vi "Addon.Version.Upgrade.vi"(8 "error in (no error)":errorcluster, 11 "Device Item Ref in in":T1 format="%.0x") -> (0 "error out":errorcluster, 3 "Device Item Ref out":T1 format="%.0x")   [LabVIEW 2025, in "Protection and Counter Addon Shared.lvlib"]
uses:
  Protection and Counter Addon Shared.lvlib
  <vilib>/NI VeriStand/Custom Device API/Custom Device Item Ref.ctl
  <vilib>/NI VeriStand/Custom Device API/Custom Device Channel.ctl
  <vilib>/NI VeriStand/Custom Device API/Custom Device Channel Type.ctl
  GUID Lookup.vi
  <vilib>/NI/NI VeriStand Advanced SysDef API/_SubVIs/SysDef.Search.GUID.vi
  <vilib>/NI/NI VeriStand Advanced SysDef API/_SubVIs/SysDef.Search.GUIDs.vi
  <vilib>/NI/NI VeriStand Advanced SysDef API/_SubVIs/SysDef.Search.Parent.vi
  NationalInstruments.VeriStand.SystemDefinitionAPI
  <vilib>/NI/NI VeriStand Advanced SysDef API/SysDef API/Advanced System Definition.lvlib
  <vilib>/NI VeriStand/Custom Device API/Custom Device API.lvlib
  SubModules/Frame-Protection-Support/Source/System Explorer/Protection and Counter Support System Explorer.lvlib
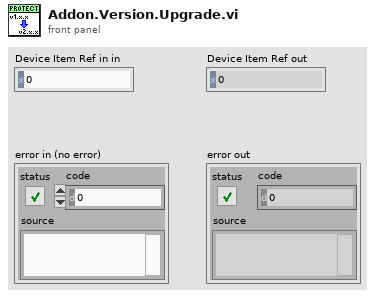
[diagram p1: front panel]
types:
  T1 = typedef "Custom Device API.lvlib/Custom Device Item Ref.ctl" = u64
  T2 = typedef "Custom Device API.lvlib/Custom Device Channel.ctl" = cluster{"Type":T3, "Units":string, "Default Value":dbl, "Faultable":bool, "Scalable":bool}
  T3 = typedef "Custom Device API.lvlib/Custom Device Channel Type.ctl" = enum16{"Input", "Output"}
  T4 = typedef "Protection and Counter Support System Explorer.lvlib/Protection Signal Settings.ctl" = cluster{"Input Channels":T5[], "Protection Type":T6}
  T5 = typedef "Protection and Counter Support System Explorer.lvlib/Protection Signal Linked Channel.ctl" = cluster{"Node Ref":T1}
  T6 = typedef "Protection and Counter Support Shared.lvlib/Protection Type.ctl" = enum16{"Arb ID + Bytes Checksum with Inversion", "Arb ID + Bytes CRC with Inversion", "Reversed Raw Signal Checksum with Inversion", "Concatenated Two's Compliment"}
  T7 = typedef "Advanced System Definition.lvlib/TreeItem.Info.ctl" = cluster{"Name":string, "Description":string, "GUID":string, "Is Channel":bool, "Channel":T2, "Is Waveform":bool, "Waveform":T8}
  T8 = typedef "Custom Device API.lvlib/Custom Device Waveform.ctl" = cluster{"Data Type":T9, "Units":string}
  T9 = typedef "Custom Device API.lvlib/Custom Device Waveform DataType.ctl" = enum16{"Double", "Complex Double"}
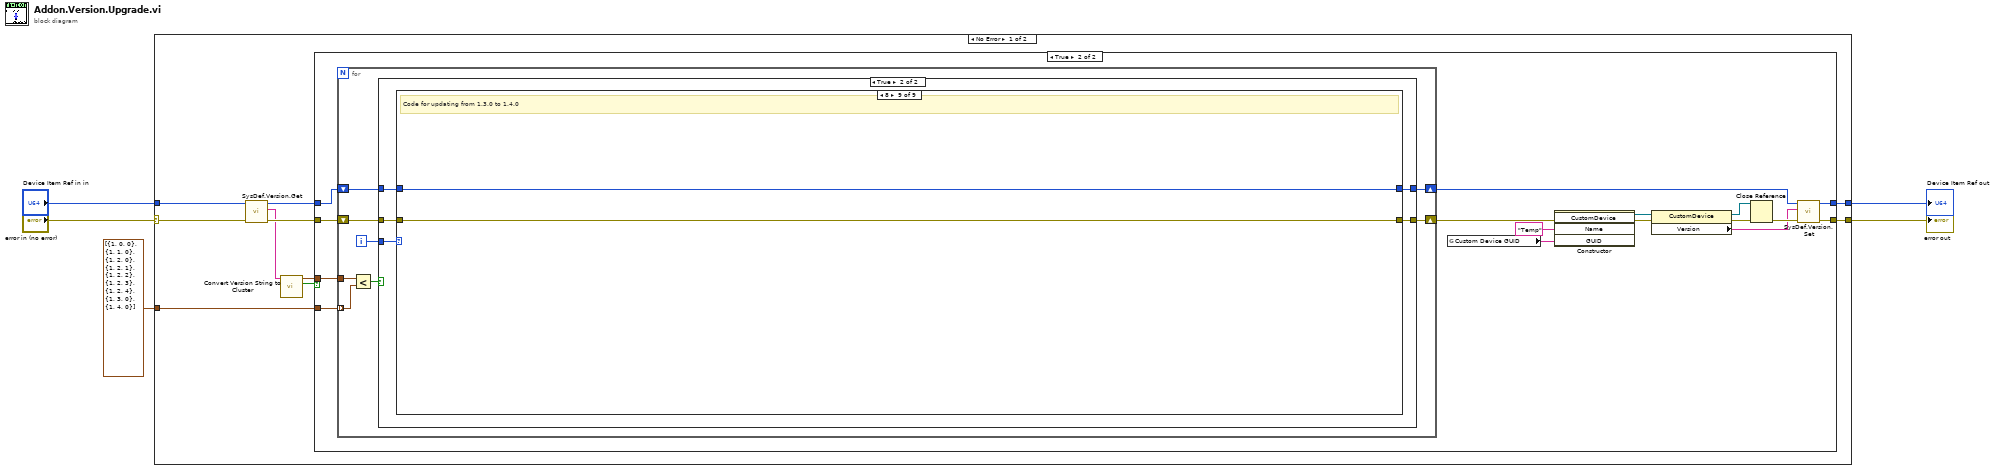
[diagram p0: block diagram]
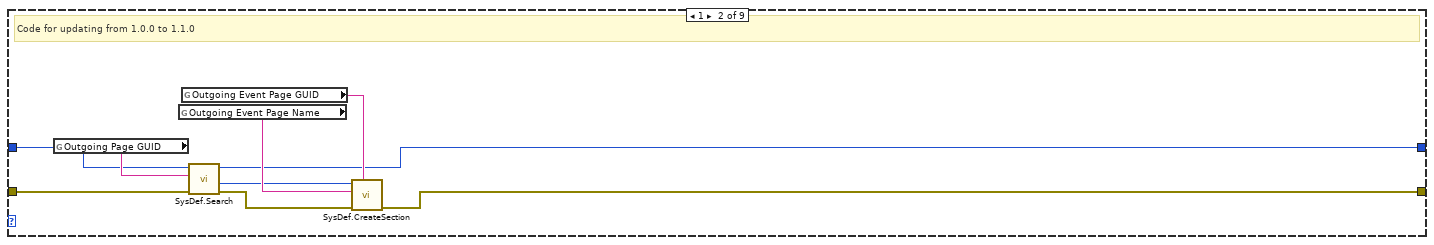
[diagram p5: hidden frame]
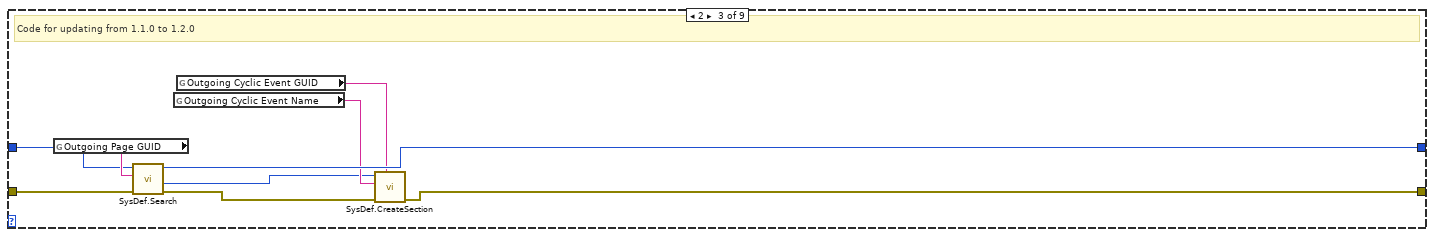
[diagram p6: hidden frame]
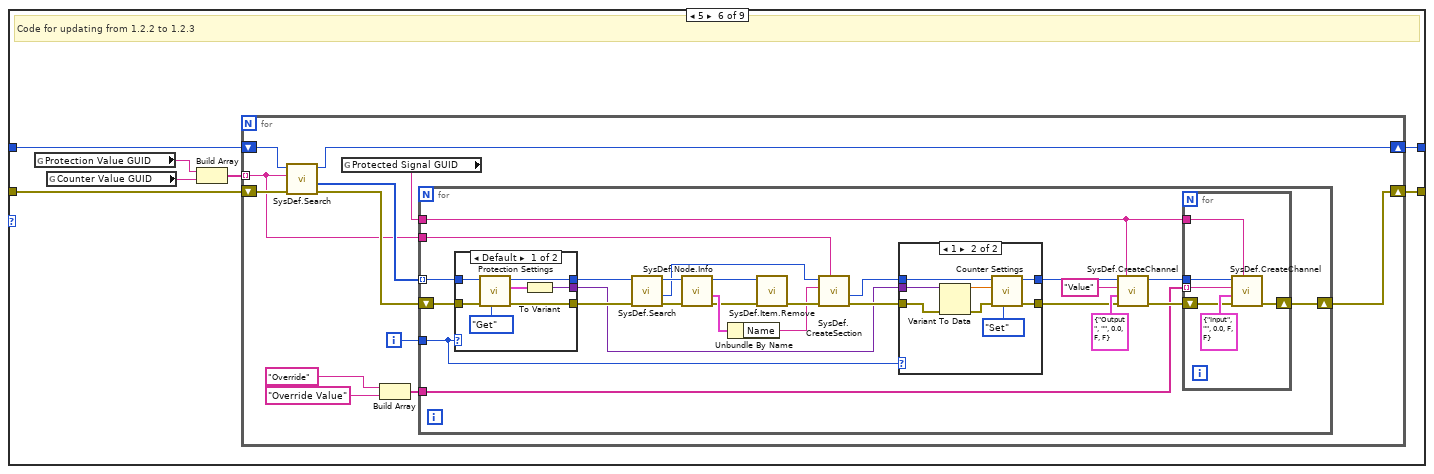
[diagram p9: hidden frame]
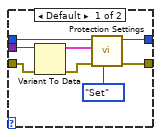
[diagram p10: hidden frame]
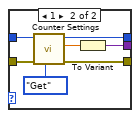
[diagram p11: hidden frame]
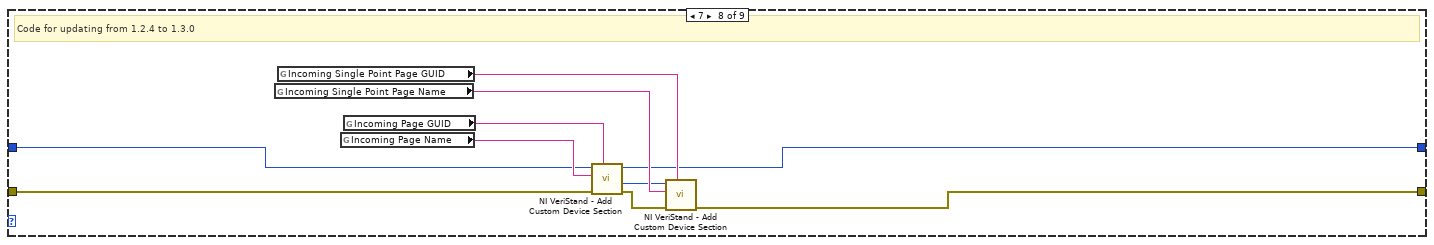
[diagram p13: hidden frame]
diagram:
  n1 = case shown="No Error" "error in (no error)" {
    selector: "error in (no error)" -> [w12 w169]
    tunnel: [w14 w169] -> w2
    tunnel: "Device Item Ref in in" -> [w11 w168]
    tunnel: [w13 w168] -> w4
    tunnel: cluster{i32, i32, i32}[] [{1, 0, 0}, {1, 1, 0}, {1, 2, 0}, {1, 2, 1}, {1, 2, 2}, {1, 2, 3}, {1, 2, 4}, {1, 3, 0}, {1, 4, 0}] -> [w15 _]
    frame No Error {
      n2 = call <vilib>:"SysDef.Version.Get.vi"("error in (no error)"=w12, "nodeID"=w11) -> ("error out"=w10:errorcluster, "Version"=w8:string, "nodeID out"=w9:u64)  [unwired: 7 in]
      n3 = call "Convert Version String to Cluster.vi"("Version"=w8) -> ("Version Valid?"=w6:bool, "Version"=w7:cluster{i32, i32, i32})  [unwired: 9 in]
      n4 = case shown="True" w6 {
        tunnel: w15 -> [_ w25]
        tunnel: [w16 w23] -> w14
        tunnel: [w17 w21] -> w13
        tunnel: w10 -> [w16 w20]
        tunnel: w9 -> [w17 w19]
        tunnel: w7 -> [_ w18]
        frame False {
        }
        frame True {
          n5 = for {
            tunnel: w25 -> [w36] mode=indexing
            shift-right: [w40] -> w24
            shift-left: w20 -> [w34]
            shift-right: [w39] -> w26
            shift-left: w19 -> [w35]
            tunnel: w18 -> [w37]
            i -> [w38]
            n6 = Less?(x=w37, y=w36) -> (x < y?=w41:bool)
            n7 = case shown="True" w41 {
              tunnel: w34 -> [w43 w48]
              tunnel: w35 -> [w42 w47]
              tunnel: [w43 w45] -> w40
              tunnel: [w42 w46] -> w39
              tunnel: w38 -> [_ w44]
              frame False {
              }
              frame True {
                n8 = case shown="8" w44 {
                  tunnel: w48 -> [w49 w56 w67 w69 w71 w78 w154 w158 w167]
                  tunnel: w47 -> [w50 w55 w66 w70 w72 w73 w155 w159 w166]
                  tunnel: [w50 w52 w65 w70 w72 w79 w155 w157 w166] -> w46
                  tunnel: [w49 w51 w62 w69 w71 w77 w154 w156 w167] -> w45
                  frame Default {
                  }
                  frame 1 {
                    # "Code for updating from 1.0.0 to 1.1.0"
                    n9 = global read "GUID Lookup.vi" "Outgoing Page GUID"() -> (w57:string)
                    n10 = global read "GUID Lookup.vi" "Outgoing Event Page Name"() -> (w59:string)
                    n11 = global read "GUID Lookup.vi" "Outgoing Event Page GUID"() -> (w58:string)
                    n12 = call-poly <vilib>:"SysDef.Search.vi"("error in (no error)"=w56, "GUID"=w57, "nodeID"=w55) -> ("error out"=w54:errorcluster, "Value out"=w53:u64, "nodeID out"=w52:u64)  [unwired: 5 in, 1 out]
                    n13 = call <vilib>:"SysDef.CreateSection.vi"("GUID"=w58, "error in (no error)"=w54, "Name"=w59, "nodeID"=w53) -> ("error out"=w51:errorcluster)  [unwired: 4 in, 3 out]
                  }
                  frame 2 {
                    # "Code for updating from 1.1.0 to 1.2.0"
                    n14 = global read "GUID Lookup.vi" "Outgoing Page GUID"() -> (w68:string)
                    n15 = call-poly <vilib>:"SysDef.Search.vi"("error in (no error)"=w67, "GUID"=w68, "nodeID"=w66) -> ("error out"=w61:errorcluster, "Value out"=w60:u64, "nodeID out"=w65:u64)  [unwired: 5 in, 1 out]
                    n16 = global read "GUID Lookup.vi" "Outgoing Cyclic Event Name"() -> (w64:string)
                    n17 = global read "GUID Lookup.vi" "Outgoing Cyclic Event GUID"() -> (w63:string)
                    n18 = call <vilib>:"SysDef.CreateSection.vi"("GUID"=w63, "error in (no error)"=w61, "Name"=w64, "nodeID"=w60) -> ("error out"=w62:errorcluster)  [unwired: 4 in, 3 out]
                  }
                  frame 3 {
                    # "Code for updating from 1.2.0 to 1.2.1"
                  }
                  frame 4 {
                    # "Code for updating from 1.2.1 to 1.2.2"
                  }
                  frame 5 {
                    # "Code for updating from 1.2.2 to 1.2.3"
                    n19 = global read "GUID Lookup.vi" "Protection Value GUID"() -> (w76:string)
                    n20 = global read "GUID Lookup.vi" "Counter Value GUID"() -> (w75:string)
                    n21 = Build Array(w76, w75) -> (w74:string[])
                    n22 = for {
                      shift-right: [w91] -> w79
                      shift-left: w73 -> [w90]
                      shift-right: [w86] -> w77
                      shift-left: w78 -> [w89]
                      tunnel: w74 -> [w81] mode=indexing
                      i -> [w80]
                      n23 = call-poly <vilib>:"SysDef.Search.vi"("error in (no error)"=w89, "GUID"=w81, "nodeID"=w90) -> ("error out"=w87:errorcluster, "Values Out"=w88:u64[], "nodeID out"=w91:u64)  [unwired: 5 in, 1 out]
                      n24 = global read "GUID Lookup.vi" "Protected Signal GUID"() -> (w82:string)
                      n25 = Build Array("Override" ("Override Name"), "Override Value" ("Override Value Name")) -> (w83:string[])
                      n26 = for {
                        tunnel: w88 -> [w98] mode=indexing
                        shift-right: [w115] -> w86
                        shift-left: w87 -> [w101]
                        tunnel: w83 -> [w114]
                        tunnel: w82 -> [w112]
                        tunnel: w81 -> [w105]
                        tunnel: w80 -> [w92]
                        n27 = case shown="Default" w92 {
                          tunnel: w101 -> [w138 w146]
                          tunnel: [w137 w145] -> w100
                          tunnel: [w136 w144] -> w99
                          tunnel: w98 -> [w139 w143]
                          tunnel: [w134 w141] -> w93
                          frame Default {
                            n28 = call "Protection Settings.vi"("Action"=enum8{"Get", "Set"}."Get", "error in"=w138, "Parent Ref"=w139) -> ("error out"=w137:errorcluster, "Selected Channels"=w135:T4, "Parent Ref Out"=w136:T1)  [unwired: 6 in]
                            n29 = To Variant(anything=w135) -> (Variant=w134:variant)
                          }
                          frame 1 {
                            n30 = call "Counter Settings.vi"("Action"=enum8{"Get", "Set"}."Get", "error in"=w146, "Parent Ref"=w143) -> ("error out"=w145:errorcluster, "Max Count"=w142:dbl, "Parent Ref Out"=w144:T1)  [unwired: 6 in]
                            n31 = To Variant(anything=w142) -> (Variant=w141:variant)
                          }
                        }
                        n32 = call-poly <vilib>:"SysDef.Search.vi"("error in (no error)"=w100, "nodeID"=w99) -> ("error out"=w104:errorcluster, "Value out"=w102:u64, "nodeID out"=w103:u64)  [unwired: 6 in, 1 out]
                        n33 = call <vilib>:"SysDef.Node.Info.vi"("error in (no error)"=w104, "nodeID"=w103) -> ("error out"=w108:errorcluster, "Item Info"=w110:T7, "nodeID out"=w109:u64)  [unwired: 6 in, 1 out]
                        n34 = Unbundle By Name(w110) -> ("Name"=w106:string)
                        n35 = call <vilib>:"SysDef.Item.Remove.vi"("error in (no error)"=w108, "nodeID"=w109) -> ("error out"=w107:errorcluster)  [unwired: 8 in, 1 out]
                        n36 = call <vilib>:"SysDef.CreateSection.vi"("GUID"=w105, "error in (no error)"=w107, "Name"=w106, "nodeID"=w102) -> ("error out"=w97:errorcluster, "New NodeID"=w95:u64)  [unwired: 4 in, 2 out]
                        n37 = case shown="1" w92 {
                          tunnel: w97 -> [w119 w127]
                          tunnel: [w122 w132] -> w96
                          tunnel: w95 -> [w124 w131]
                          tunnel: [w123 w130] -> w94
                          tunnel: w93 -> [w121 w129]
                          frame Default {
                            n38 = Variant To Data(error in=w119, Variant=w121) -> (data=w118:T4, error out=w120:errorcluster)  [unwired: 1 in]
                            n39 = call "Protection Settings.vi"("Action"=enum8{"Get", "Set"}."Set", "error in"=w120, "Selected Channels"=w118, "Parent Ref"=w124) -> ("error out"=w122:errorcluster, "Parent Ref Out"=w123:T1)  [unwired: 5 in, 1 out]
                          }
                          frame 1 {
                            n40 = Variant To Data(error in=w127, Variant=w129) -> (data=w126:dbl, error out=w128:errorcluster)  [unwired: 1 in]
                            n41 = call "Counter Settings.vi"("Action"=enum8{"Get", "Set"}."Set", "error in"=w128, "Max Count"=w126, "Parent Ref"=w131) -> ("error out"=w132:errorcluster, "Parent Ref Out"=w130:T1)  [unwired: 5 in, 1 out]
                          }
                        }
                        n42 = call <vilib>:"SysDef.CreateChannel.vi"("GUID"=w112, "error in (no error)"=w96, "Channel"=T2 {"Type"=enum."Output", "Units"="", "Default Value"=0.0, "Faultable"=FALSE, "Scalable"=FALSE}, "Name"="Value" ("Override Name"), "nodeID"=w94) -> ("error out"=w116:errorcluster, "nodeID out"=w113:u64)  [unwired: 3 in, 2 out]
                        n43 = for {
                          tunnel: w114 -> [w150] mode=indexing
                          tunnel: w113 -> [w149]
                          tunnel: w112 -> [w148]
                          shift-right: [w151] -> w115
                          shift-left: w116 -> [w152]
                          n44 = call <vilib>:"SysDef.CreateChannel.vi"("GUID"=w148, "error in (no error)"=w152, "Channel"=T2 {"Type"=enum."Input", "Units"="", "Default Value"=0.0, "Faultable"=FALSE, "Scalable"=FALSE}, "Name"=w150, "nodeID"=w149) -> ("error out"=w151:errorcluster)  [unwired: 3 in, 3 out]
                        }
                      }
                    }
                  }
                  frame 6 {
                    # "Code for updating from 1.2.3 to 1.2.4"
                  }
                  frame 7 {
                    # "Code for updating from 1.2.4 to 1.3.0"
                    n45 = global read "GUID Lookup.vi" "Incoming Single Point Page Name"() -> (w162:string)
                    n46 = global read "GUID Lookup.vi" "Incoming Single Point Page GUID"() -> (w163:string)
                    n47 = global read "GUID Lookup.vi" "Incoming Page Name"() -> (w164:string)
                    n48 = global read "GUID Lookup.vi" "Incoming Page GUID"() -> (w165:string)
                    n49 = call <vilib>:"NI VeriStand - Add Custom Device Section.vi"("GUID (Default Section)"=w165, "error in (no error)"=w158, "Section Name"=w164, "Parent Ref in"=w159) -> ("error out"=w160:errorcluster, "Section Ptr"=w161:T1, "Parent Ref out"=w157:T1)  [unwired: 4 in, 1 out]
                    n50 = call <vilib>:"NI VeriStand - Add Custom Device Section.vi"("GUID (Default Section)"=w163, "error in (no error)"=w160, "Section Name"=w162, "Parent Ref in"=w161) -> ("error out"=w156:errorcluster)  [unwired: 4 in, 3 out]
                  }
                  frame 8 {
                    # "Code for updating from 1.3.0 to 1.4.0"
                  }
                }
              }
            }
          }
          n51 = global read "GUID Lookup.vi" "Custom Device GUID"() -> (w22:string)
          n52 = constructor class="CustomDevice"(error in=w24, "Name"="Temp", "GUID"=w22) -> (reference out=w33:refnum<k24>, error out=w32:errorcluster)  [unwired: 2 in, 3 out]
          n53 = property class="CustomDevice"(reference=w33, error in=w32) -> (reference out=w30:refnum<k24>, error out=w31:errorcluster, "Version"=w28:string)
          n54 = Close Reference(reference=w30, error in (no error)=w31) -> (error out=w29:errorcluster)
          n55 = call <vilib>:"SysDef.Version.Set.vi"("error in (no error)"=w29, "Version"=w28, "nodeID"=w26) -> ("error out"=w23:errorcluster, "nodeID out"=w21:u64)  [unwired: 7 in]
        }
      }
    }
    frame Error {
    }
  }
  "Device Item Ref out" <- w4
  "error out" <- w2
